vi "RI_OPEN.vi"(2 "error in (no error)":errorcluster, 3 "Cluster":T2) -> (0 "error out":errorcluster, 1 "output cluster":T1)   [LabVIEW 2021]
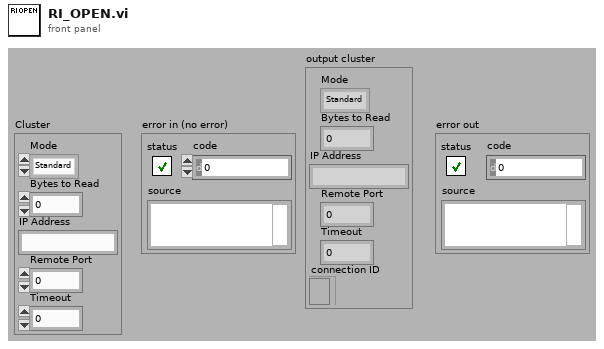
[diagram p1: front panel]
types:
  T1 = cluster{"Mode":enum16{"Standard", "Buffered", "CRLF", "Immediate"}, "Bytes to Read":i32, "IP Address":string, "Remote Port":i32, "Timeout":i32, "connection ID":refnum<k5>}
  T2 = cluster{"Mode":enum16{"Standard", "Buffered", "CRLF", "Immediate"}, "Bytes to Read":i32, "IP Address":string, "Remote Port":i32, "Timeout":i32}
  T3 = enum16{"Standard", "Buffered", "CRLF", "Immediate"}
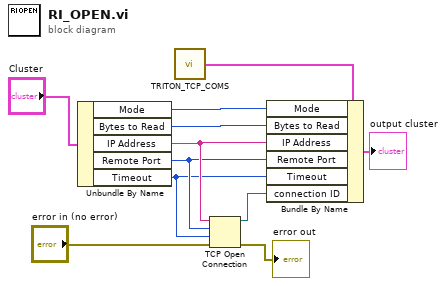
[diagram p0: block diagram]
diagram:
  n1 = Unbundle By Name("Cluster") -> ("Mode"=w6:T3, "Bytes to Read"=w5:i32, "IP Address"=w4:string, "Remote Port"=w3:i32, "Timeout"=w2:i32)
  n2 = call "TRITON_TCP_COMS.vi"() -> ("Cluster"=w8:T1)
  n3 = TCP Open Connection(address=w4, remote port or service name=w3, timeout ms (60000)=w2, error in (no error)="error in (no error)") -> (connection ID=w7:refnum<k5>, error out=→"error out":errorcluster)  [unwired: 1 in]
  n4 = Bundle By Name(cluster=w8, "Mode"=w6, "Bytes to Read"=w5, "IP Address"=w4, "Remote Port"=w3, "Timeout"=w2, "connection ID"=w7) -> (→"output cluster":T1)
